vi "DRIVE_SPEED_CONTROL.vi"(4 "Time_Seconds":dbl, 5 "Speed PID":T2, 6 "Speed (PV)":dbl, 7 "SIMPLE_MOTOR_FF":T1 {"Ka" format="%13.4f"; "Kv" format="%13.4f"; "Ks" format="%13.4f"}, 9 "Speed Target (SP)":dbl, 10 "Max SP Rate":dbl, 11 "Max Speed Ft/Sec":dbl) -> (0 "FeedForward":dbl, 1 "SpeedDmdAccel":dbl, 2 "SpeedDmd":dbl, 3 "CO-ControlOutput":dbl)   [LabVIEW 2019]
uses:
  <vilib>/Rock Robotics/WPI/ThirdParty/JAS_Junk/TrajLib/Trajectory_Library.lvlib
  <vilib>/Rock Robotics/WPI/ThirdParty/JAS_Junk/TrajLib/SIMPLE_MOTOR_FF.ctl
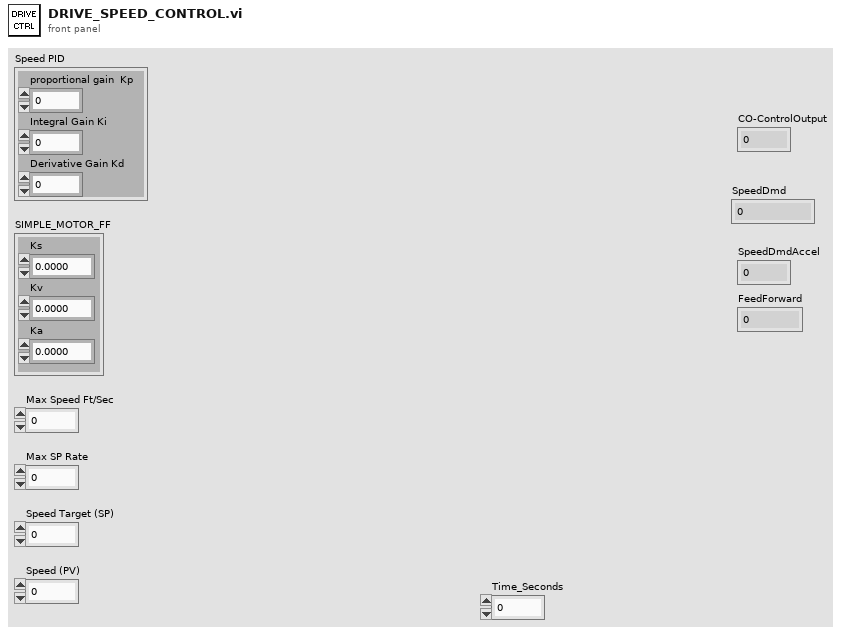
[diagram p1: front panel]
types:
  T1 = typedef "Trajectory_Library.lvlib/SIMPLE_MOTOR_FF.ctl" = cluster{"Ks":dbl, "Kv":dbl, "Ka":dbl}
  T2 = cluster{"proportional gain  Kp":dbl, "Integral Gain Ki":dbl, "Derivative Gain Kd":dbl}
  T3 = typedef "Trajectory_Library.lvlib/PID_ADV_TUNING.ctl" = cluster{"Kf":dbl, "Kp":dbl, "Ki":dbl, "Kd":dbl, "MaximumIntegral":dbl, "MinimumIntegral":dbl, "Filter Derivative":bool}
  T4 = typedef "Trajectory_Library.lvlib/PID_ADV_LIMITS.ctl" = cluster{"MaxInput":dbl, "MinInput":dbl, "Continuous":bool, "MaxOutput":dbl, "MinOutput":dbl}
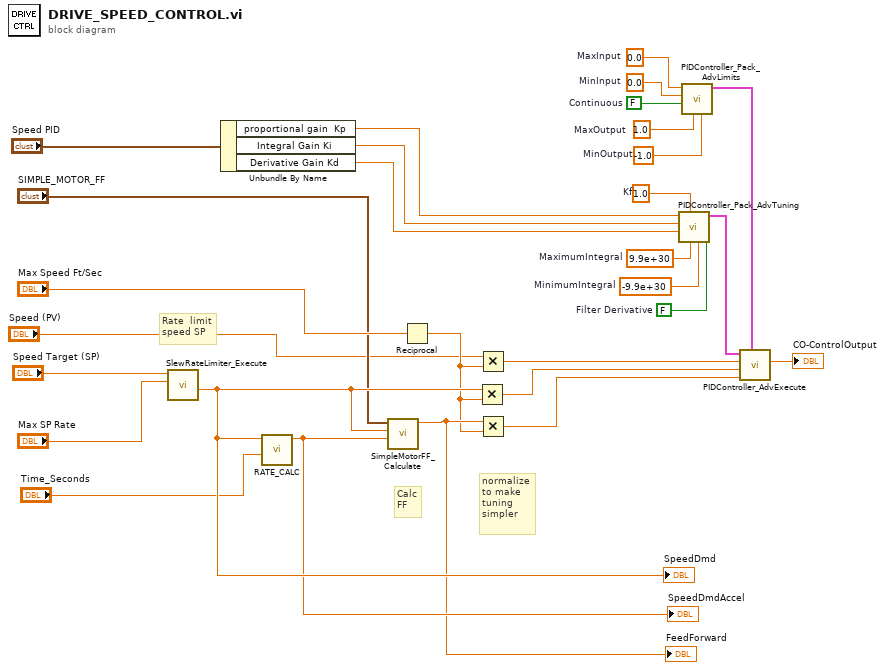
[diagram p0: block diagram]
diagram:
  w10 = 1.0  # Kf
  w11 = 9.9e+30  # MaximumIntegral
  w12 = -9.9e+30  # MinimumIntegral
  w13 = FALSE  # Filter Derivative
  w15 = 0.0  # MinInput
  w16 = FALSE  # Continuous
  w17 = 1.0  # MaxOutput
  w14 = -1.0  # MinOutput
  w18 = 0.0  # MaxInput
  # "Calc\nFF"
  # "Rate  limit\nspeed SP"
  # "normalize\nto make\ntuning\nsimpler"
  n1 = call <vilib>:"SlewRateLimiter_Execute.vi"("Rate"="Max SP Rate", "Input"="Speed Target (SP)") -> ("Output"=w29:dbl)  [unwired: 8 in, 1 out]
  "SpeedDmd" <- w29
  n2 = Unbundle By Name("Speed PID") -> ("proportional gain  Kp"=w25:dbl, "Integral Gain Ki"=w26:dbl, "Derivative Gain Kd"=w27:dbl)
  n3 = call "RATE_CALC.vi"("Time"="Time_Seconds", "Input"=w29) -> ("Output"=w8:dbl)  [unwired: 9 in]
  "SpeedDmdAccel" <- w8
  n4 = call <vilib>:"SimpleMotorFF_Calculate.vi"("Accel"=w8, "Vel"=w29, "SIMPLE_MOTOR_FF"="SIMPLE_MOTOR_FF") -> ("FeedForward"=w5:dbl)  [unwired: 8 in]
  "FeedForward" <- w5
  n5 = Reciprocal(x="Max Speed Ft/Sec") -> (1/x=w4:dbl)
  n6 = Multiply(x=w29, y=w4) -> (x*y=w21:dbl)
  n7 = Multiply(x="Speed (PV)", y=w4) -> (x*y=w24:dbl)
  n8 = Multiply(x=w5, y=w4) -> (x*y=w22:dbl)
  n9 = call <vilib>:"PIDController_Pack_AdvTuning.vi"("Filter Derivative"=w13, "MinimumIntegral"=w12, "MaximumIntegral"=w11, "Kf"=w10, "Kd"=w27, "Ki"=w26, "Kp"=w25) -> ("Adv PID Tuning"=w19:T3)  [unwired: 4 in]
  n10 = call <vilib>:"PIDController_Pack_AdvLimits.vi"("MinOutput"=w14, "MaxOutput"=w17, "Continuous"=w16, "MinInput"=w15, "MaxInput"=w18) -> ("Adv PID Limits"=w20:T4)  [unwired: 6 in]
  n11 = call <vilib>:"PIDController_AdvExecute.vi"("Adv PID Limits"=w20, "FF-FeedForward"=w22, "SP-SetPoint"=w21, "PV-Measurement"=w24, "Adv PID Tuning"=w19) -> ("CO-ControlOutput"=→"CO-ControlOutput":dbl)  [unwired: 4 in, 2 out]
